vi "TEST_plot_boat.vi"() -> ()   [LabVIEW 2013]
uses:
  cRIO_Code/Data/TypeDefs/UTM Location.ctl
  cRIO_Code/Data/TypeDefs/Sail Set Suggestions.ctl
  cRIO_Code/Data/TypeDefs/Rudder Set Suggestions.ctl
panel:
  in  "Rudder Setpoint":T1 min=-0.95 max=0.95 scale=1.0..-1.0
  in  "Sail Setpoints":T2 {"MainSailSuggestion" min=0.0 max=1.0; "JibSailSuggestion" min=0.0 max=1.0}
  in  "Map":enum16{"Grid"}(ring)
  in  "Trace Path":bool=TRUE
  out "Boat Outside Img":bool
  in  "Heading":dbl
  in  "stop":bool
  in  "UTM boat location":T3={"UTM Zone"=0.0, "Hemisphere"=enum."North", "East"=1.0, "North"=1.0} {"North" format="%#_10f"; "East" format="%#_8f"}
  out "Mission Map":T4(plugin-control)
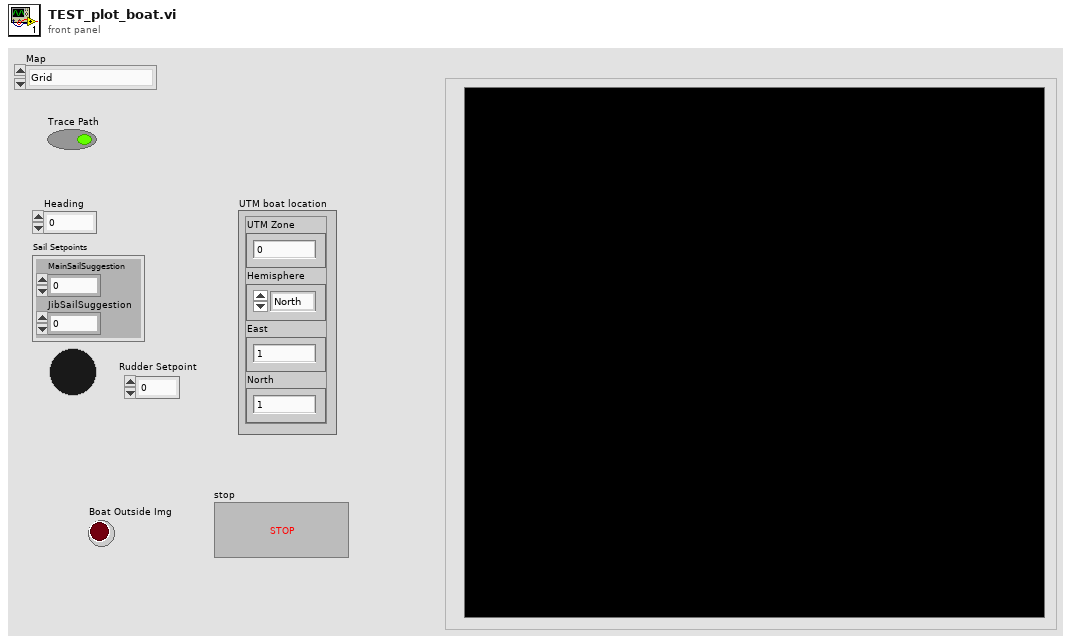
[diagram p1: front panel]
types:
  T1 = typedef "Rudder Set Suggestions.ctl" = dbl
  T2 = typedef "Sail Set Suggestions.ctl" = cluster{"MainSailSuggestion":dbl, "JibSailSuggestion":dbl}
  T3 = typedef "UTM Location.ctl" = cluster{"UTM Zone":dbl, "Hemisphere":enum16{"North", "South"}, "East":dbl, "North":dbl}
  T4 = typedef "IMAQ Image.ctl" = refnum<image>
  T5 = typedef "MapDistanceInfo.ctl" = cluster{"Meters/pixel":dbl, "Top Left Pixel UTM":T3, "Bottom Right Pixel UTM":T3}
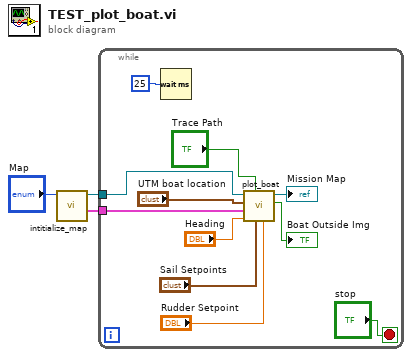
[diagram p0: block diagram]
diagram:
  n1 = call "intitialize_map.vi"("Map"="Map") -> ("MapDistanceInfo"=w2:T5, "Map Image Out"=w3:T4)  [unwired: 9 in]
  n2 = while {
    tunnel: w3 -> [w14]
    tunnel: w2 -> [w7]
    stop <- "stop" stop-if-true
    n3 = Wait (ms)(milliseconds to wait=u32 25) -> ()  [unwired: 1 out]
    n4 = call "plot_boat.vi"("Rudder Setpoint"="Rudder Setpoint", "Sail Setpoints"="Sail Setpoints", "Trace Path"="Trace Path", "Heading"="Heading", "MapDistanceInfo"=w7, "UTM Location"="UTM boat location", "Map in"=w14) -> ("Boat Outside Img"=→"Boat Outside Img":bool, "Map Out"=→"Mission Map":T4)  [unwired: 2 in, 1 out]
  }
